vi "spi_8bit.vi"(9 "Hex":i8 format="%02x", 11 "I/O Cluster In":T1) -> (3 "I/O Cluster Out":T1)   [LabVIEW 2016, in "jmslib.lvlib"]
uses:
  jmslib.lvlib
  KevinLibraryAll/labview2010/kevLib2010.lvlib
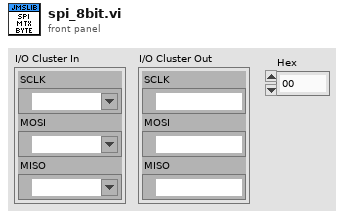
[diagram p1: front panel]
types:
  T1 = cluster{"SCLK":refnum<k21>, "MOSI":refnum<k21>, "MISO":refnum<k21>}
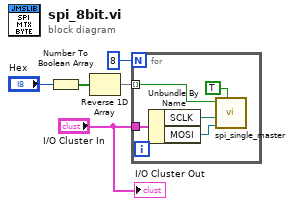
[diagram p0: block diagram]
diagram:
  n1 = Number To Boolean Array(number="Hex") -> (Boolean array=w3:bool[])
  n2 = Reverse 1D Array(array=w3) -> (reversed array=w2:bool[])
  n3 = for {
    N: 8 -> [_]
    tunnel: w2 -> [w9] mode=indexing
    tunnel: "I/O Cluster In" -> [w8]
    n4 = Unbundle By Name(w8) -> ("SCLK"=w7:refnum<k21>, "MOSI"=w6:refnum<k21>)
    n5 = call "spi_single_master.vi"("Falling Edge?"=TRUE, "SIG Port"=w6, "CLK Port"=w7, "Signal"=w9) -> ()  [unwired: 6 in, 2 out]
  }
  "I/O Cluster Out" <- "I/O Cluster In"
